vi "Test Create and Add Instrument1.vi"(11 "Test Case In":refnum<class "Measure and Stimulus Subsystems.lvclass">) -> (0 "error out":errorcluster, 3 "Test Case Out":refnum<class "Measure and Stimulus Subsystems.lvclass">)   [LabVIEW 2023, in "Measure and Stimulus Subsystems.lvclass"]
uses:
  Measure and Stimulus Subsystems.lvclass
  C:/Program Files/National Instruments/LabVIEW 2023/vi.lib/Astemes/LUnit/Test Case.lvclass
  Measure and Stimulus Subsystems/Measure and Stimulus Subsystems.lvclass
  Devices/Red-y/Configurations/Pressure Control CFG Simulated/Red-y Pressure Control CFG Simulated.lvclass
  AO/AO DAQmx DC Simulated CFG/AO DAQmx DC Simulated CFG.lvclass
  <vilib>/Astemes/LUnit/Test Case.lvclass/Test Case.ctl
  4993e8ee-a06a-463a-9684-69129f64d5ce.vi
  <vilib>/Astemes/LUnit/Append Pass Result.vi
  <vilib>/Astemes/LUnit/Append Fail Result.vi
  <vilib>/Astemes/LUnit/Describe Comparison.vi
  <vilib>/Astemes/LUnit/Compare Variants.vi
  <vilib>/Astemes/LUnit/Run In UI.vi
  <vilib>/Utility/error.llb/Clear Errors.vi
  <vilib>/Astemes/LUnit/Describe Variant.vi
  Measure and Stimulus Subsystems.lvclass/Measure and Stimulus Subsystems.ctl
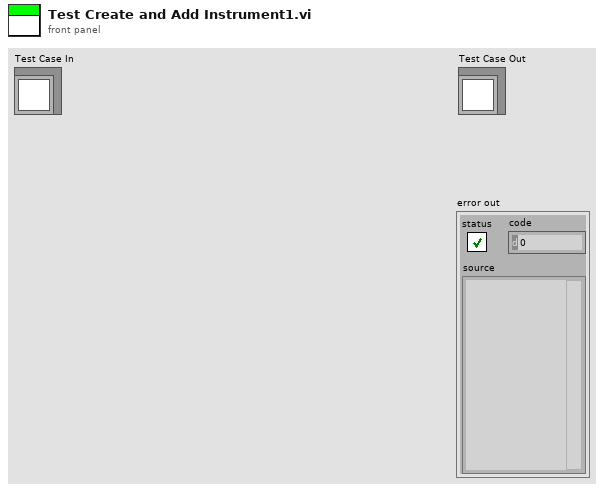
[diagram p1: front panel]
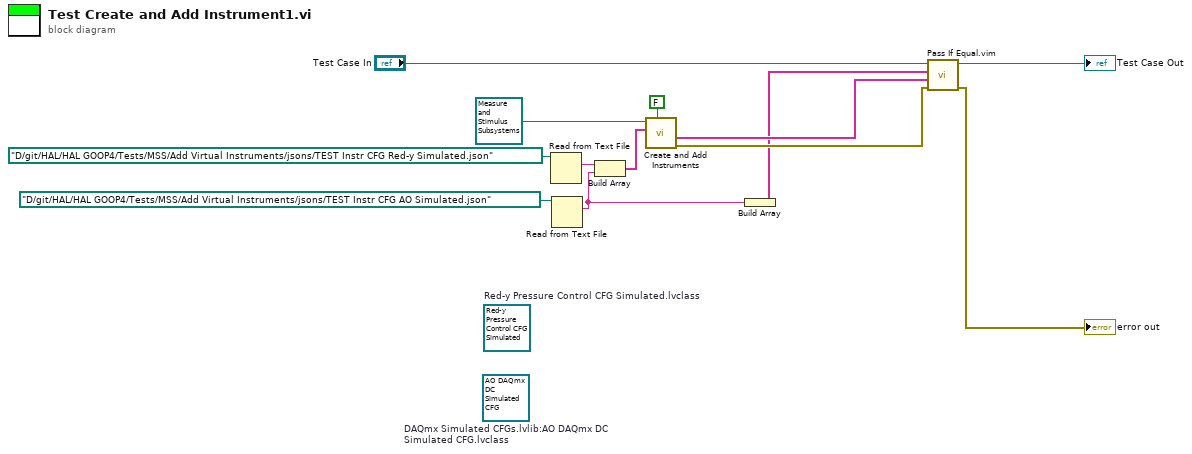
[diagram p0: block diagram]
diagram:
  (unwired) refnum<class "AO DAQmx DC Simulated CFG.lvclass"> refnum  # DAQmx Simulated CFGs.lvlib:AO DAQmx DC Simulated CFG.lvclass
  (unwired) refnum<class "Red-y Pressure Control CFG Simulated.lvclass"> refnum  # Red-y Pressure Control CFG Simulated.lvclass
  n1 = Read from Text File(file (use dialog)=path "D:/git/HAL/HAL GOOP4/Tests/MSS/Add Virtual Instruments/jsons/TEST Instr CFG Red-y Simulated.json") -> (text=w7:string)  [unwired: 3 in, 3 out]
  n2 = Read from Text File(file (use dialog)=path "D:/git/HAL/HAL GOOP4/Tests/MSS/Add Virtual Instruments/jsons/TEST Instr CFG AO Simulated.json") -> (text=w2:string)  [unwired: 3 in, 3 out]
  n3 = Build Array(w7, w2) -> (w6:string[])
  n4 = call "Create and Add Instruments.vi"("Is Target?"=FALSE, "Physical Intr CFGs"=w6, "MSS in"=refnum<class "Measure and Stimulus Subsystems.lvclass"> refnum) -> ("Error Out"=w5:errorcluster, "Target Physical Instr CFGs"=w4:string[])  [unwired: 6 in, 1 out]
  n5 = Build Array(w2) -> (w1:string[])
  n6 = call "Pass If Equal.vim"("error in (no error)"=w5, "Actual"=w4, "Expected"=w1, "LUnit Test Case In"="Test Case In") -> ("error out"=→"error out":errorcluster, "LUnit Test Case Out"=→"Test Case Out":refnum<class "Measure and Stimulus Subsystems.lvclass">)  [unwired: 6 in]
